vi "dsmm-registration.vi"(0 "X":dbl[][](array[numeric]), 1 "allocate":bool=TRUE, 2 "allocate_size":i32=90000, 3 "gamma0":dbl=0.1, 5 "Y":dbl[][](array[numeric]), 7 "beta":dbl=3.0, 9 "lambda":dbl=1.0, 11 "neighbor_cutoff":dbl=10.0, 12 "alpha":dbl=1.0, 13 "conv_epsilon":dbl=0.0001, 14 "eq_tol":dbl=0.001) -> (4 "X out":dbl[][](array[numeric]), 6 "Y out":dbl[][](array[numeric]), 8 "Match":i32[](array[numeric]), 10 "p":dbl[][](array[numeric]))   [LabVIEW 2017]
uses:
  dll/wormUtilities/x64/Release/wormUtilities.dll
panel:
  # "Registers Y onto X"
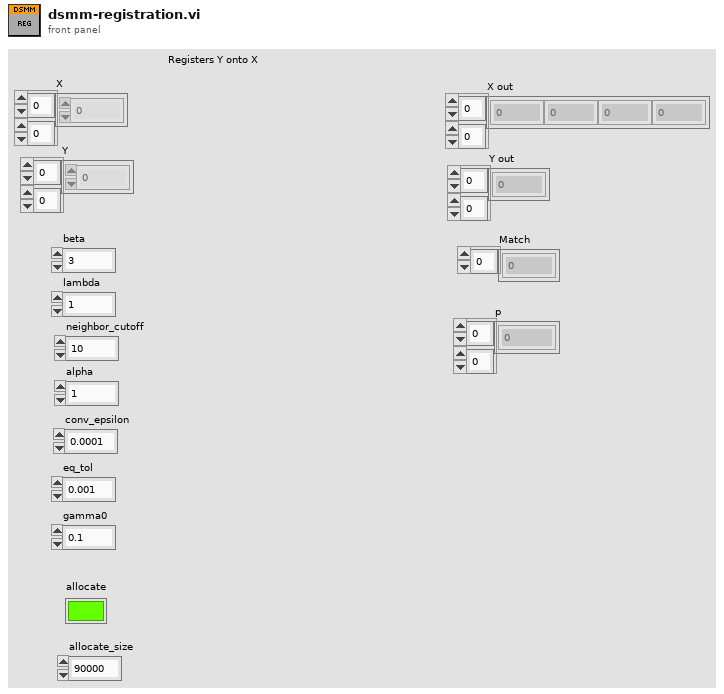
[diagram p1: front panel]
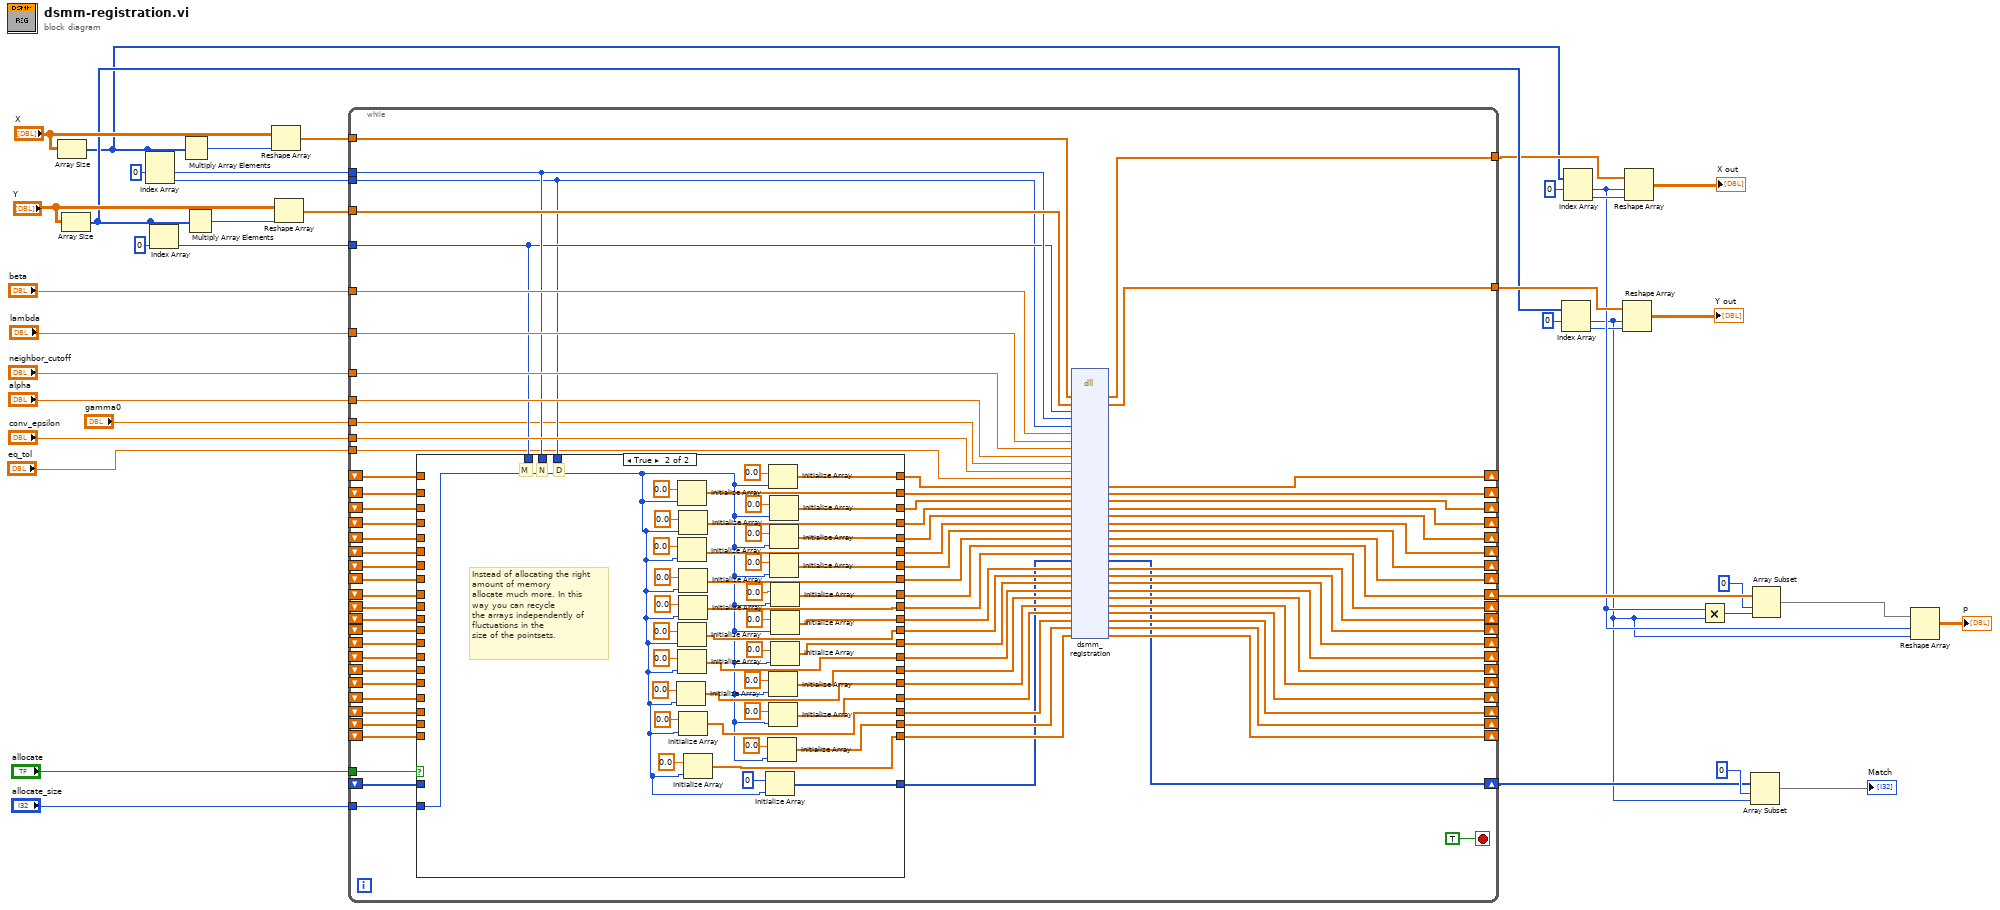
[diagram p0: block diagram]
diagram:
  n1 = Array Size(array="X") -> (size(s)=w10:i32[])
  n2 = Array Size(array="Y") -> (size(s)=w16:i32[])
  n3 = Index Array(array=w10, index #1=0 ("index")) -> (element #1=w31:i32, element #2=w30:i32)  [unwired: 1 in]
  n4 = Index Array(array=w16, index=0) -> (element=w25:i32)
  n5 = Multiply Array Elements(1:w10) -> (0:w33:i32)
  n6 = Multiply Array Elements(1:w16) -> (0:w29:i32)
  n7 = Reshape Array("X", w33) -> (w32:dbl[])
  n8 = Reshape Array("Y", w29) -> (w26:dbl[])
  n9 = while {
    tunnel: "beta" -> [w120]
    tunnel: "lambda" -> [w119]
    tunnel: "neighbor_cutoff" -> [w118]
    tunnel: "alpha" -> [w117]
    tunnel: "conv_epsilon" -> [w116]
    tunnel: [w115] -> w21
    tunnel: w32 -> [w113]
    tunnel: w31 -> [w51]
    tunnel: w30 -> [w49]
    tunnel: w26 -> [w112]
    tunnel: w25 -> [w50]
    shift-right: [w111] -> _
    shift-left: _ -> [w92]
    shift-right: [w110] -> _
    shift-left: _ -> [w90]
    shift-right: [w109] -> _
    shift-left: _ -> [w88]
    shift-right: [w108] -> _
    shift-left: _ -> [w87]
    shift-right: [w107] -> _
    shift-left: _ -> [w85]
    shift-right: [w106] -> _
    shift-left: _ -> [w84]
    shift-right: [w105] -> _
    shift-left: _ -> [w80]
    shift-right: [w104] -> _
    shift-left: _ -> [w78]
    shift-right: [w114] -> w19
    shift-left: _ -> [w76]
    shift-right: [w103] -> _
    shift-left: _ -> [w74]
    shift-right: [w102] -> _
    shift-left: _ -> [w72]
    shift-right: [w101] -> _
    shift-left: _ -> [w70]
    shift-right: [w100] -> _
    shift-left: _ -> [w68]
    shift-right: [w99] -> _
    shift-left: _ -> [w66]
    shift-right: [w98] -> _
    shift-left: _ -> [w64]
    shift-right: [w97] -> _
    shift-left: _ -> [w62]
    shift-right: [w96] -> _
    shift-left: _ -> [w60]
    shift-right: [w95] -> _
    shift-left: _ -> [w58]
    shift-right: [w94] -> _
    shift-left: _ -> [w56]
    shift-right: [w93] -> _
    shift-left: _ -> [w54]
    tunnel: "allocate" -> [w52]
    tunnel: "allocate_size" -> [w48]
    tunnel: [w46] -> w11
    shift-right: [w44] -> w5
    shift-left: _ -> [w43]
    tunnel: "gamma0" -> [w42]
    tunnel: "eq_tol" -> [w41]
    stop <- TRUE stop-if-true
    n10 = case shown="True" w52 {
      tunnel: w92 -> [w141 _]
      tunnel: [w141 w183] -> w91
      tunnel: w90 -> [w140 _]
      tunnel: [w140 w181] -> w89
      tunnel: w88 -> [w122 _]
      tunnel: [w122 w179] -> w81
      tunnel: w87 -> [w139 _]
      tunnel: [w139 w177] -> w86
      tunnel: w85 -> [w123 _]
      tunnel: [w123 w175] -> w82
      tunnel: w84 -> [w138 _]
      tunnel: [w138 w169] -> w83
      tunnel: w80 -> [w137 _]
      tunnel: [w137 w173] -> w79
      tunnel: [w136 w167] -> w77
      tunnel: w78 -> [w136 _]
      tunnel: [w135 w171] -> w75
      tunnel: w76 -> [w135 _]
      tunnel: [w134 w165] -> w73
      tunnel: w74 -> [w134 _]
      tunnel: [w133 w163] -> w71
      tunnel: w72 -> [w133 _]
      tunnel: w70 -> [w132 _]
      tunnel: [w132 w161] -> w69
      tunnel: w68 -> [w131 _]
      tunnel: [w131 w159] -> w67
      tunnel: w66 -> [w130 _]
      tunnel: [w130 w157] -> w65
      tunnel: w64 -> [w129 _]
      tunnel: [w129 w155] -> w63
      tunnel: w62 -> [w128 _]
      tunnel: [w128 w153] -> w61
      tunnel: w60 -> [w127 _]
      tunnel: [w127 w151] -> w59
      tunnel: w58 -> [w126 _]
      tunnel: [w126 w149] -> w57
      tunnel: w56 -> [w125 _]
      tunnel: [w125 w147] -> w55
      tunnel: w54 -> [w124 _]
      tunnel: [w124 w145] -> w53
      tunnel: w51 -> [_ _]
      tunnel: w50 -> [_ _]
      tunnel: w49 -> [_ _]
      tunnel: w48 -> [_ w142]
      tunnel: [w121 w144] -> w45
      tunnel: w43 -> [w121 _]
      frame False {
      }
      frame True {
        # "Instead of allocating the right amount of memory\nallocate much more. In this way you can recycle\nthe arrays independently of fluctuations in the \nsize of the pointsets."
        # "D"
        # "N"
        # "M"
        n11 = Initialize Array(0.0 ("element"), w142) -> (w153:dbl[])
        n12 = Initialize Array(0.0 ("element"), w142) -> (w181:dbl[])
        n13 = Initialize Array(0.0 ("element"), w142) -> (w169:dbl[])
        n14 = Initialize Array(0.0 ("element"), w142) -> (w161:dbl[])
        n15 = Initialize Array(0.0 ("element"), w142) -> (w157:dbl[])
        n16 = Initialize Array(0.0 ("element"), w142) -> (w177:dbl[])
        n17 = Initialize Array(0.0 ("element"), w142) -> (w167:dbl[])
        n18 = Initialize Array(0.0 ("element"), w142) -> (w165:dbl[])
        n19 = Initialize Array(0.0 ("element"), w142) -> (w149:dbl[])
        n20 = Initialize Array(0.0 ("element"), w142) -> (w145:dbl[])
        n21 = Initialize Array(0 ("dimension size"), w142) -> (w144:i32[])
        n22 = Initialize Array(0.0 ("element"), w142) -> (w147:dbl[])
        n23 = Initialize Array(0.0 ("element"), w142) -> (w183:dbl[])
        n24 = Initialize Array(0.0 ("element"), w142) -> (w155:dbl[])
        n25 = Initialize Array(0.0 ("element"), w142) -> (w151:dbl[])
        n26 = Initialize Array(0.0 ("element"), w142) -> (w179:dbl[])
        n27 = Initialize Array(0.0 ("element"), w142) -> (w175:dbl[])
        n28 = Initialize Array(0.0 ("element"), w142) -> (w173:dbl[])
        n29 = Initialize Array(0.0 ("element"), w142) -> (w171:dbl[])
        n30 = Initialize Array(0.0 ("element"), w142) -> (w163:dbl[])
        n31 = Initialize Array(0.0 ("element"), w142) -> (w159:dbl[])
      }
    }
    n32 = dll-call lib="C:/Users/francesco/dev/pump-probe/dll/wormUtilities/x64/Release/wormUtilities.dll" fn="dsmm_registration"("X"=w113, "Y"=w112, "M"=w50, "N"=w51, "D"=w49, "beta"=w120, "lambda"=w119, "neighbor_cutoff"=w118, "alpha"=w117, "gamma0"=w42, "conv_epsilon"=w116, "eq_tol"=w41, "pwise_dist"=w91, "pwise_distYY"=w89, "Gamma"=w81, "CDE_term"=w86, "w"=w82, "F_t"=w83, "wF_t"=w79, "wF_t_sum"=w77, "p"=w75, "u"=w73, "Match"=w45, "hatP"=w71, "hatPI_diag"=w69, "hatPIG"=w67, "hatPX"=w65, "hatPIY"=w63, "G"=w61, "W"=w59, "GW"=w57, "sumPoverN"=w55, "expAlphaSumPoverN"=w53) -> ("X"=w46:dbl[], "Y"=w115:dbl[], "pwise_dist"=w111:dbl[], "pwise_distYY"=w110:dbl[], "Gamma"=w109:dbl[], "CDE_term"=w108:dbl[], "w"=w107:dbl[], "F_t"=w106:dbl[], "wF_t"=w105:dbl[], "wF_t_sum"=w104:dbl[], "p"=w114:dbl[], "u"=w103:dbl[], "Match"=w44:i32[], "hatP"=w102:dbl[], "hatPI_diag"=w101:dbl[], "hatPIG"=w100:dbl[], "hatPX"=w99:dbl[], "hatPIY"=w98:dbl[], "G"=w97:dbl[], "W"=w96:dbl[], "GW"=w95:dbl[], "sumPoverN"=w94:dbl[], "expAlphaSumPoverN"=w93:dbl[])  [unwired: 14 in, 2 out]
  }
  n33 = Index Array(array=w16, index #1=0 ("index")) -> (element #1=w2:i32, element #2=w3:i32)  [unwired: 1 in]
  n34 = Index Array(array=w10, index #1=0 ("index")) -> (element #1=w4:i32, element #2=w13:i32)  [unwired: 1 in]
  n35 = Reshape Array(w21, w2, w3) -> (→"Y out":dbl[][])
  n36 = Reshape Array(w11, w4, w13) -> (→"X out":dbl[][])
  n37 = Multiply(x=w4, y=w2) -> (x*y=w9:i32)
  n38 = Array Subset(array=w5, index=0, length=w2) -> (→"Match":i32[])
  n39 = Array Subset(array=w19, index=0, length=w9) -> (w17:dbl[])
  n40 = Reshape Array(w17, w4, w2) -> (→"p":dbl[][])
